vi "Update Low Limit.vi"(7 "Type":T1, 8 "error in (no error)":errorcluster, 9 "Low Limit":dbl, 10 "Channel Name":string, 11 "User BluelinesRedlines in":refnum<class "User BluelinesRedlines.lvclass">) -> (0 "error out":errorcluster, 3 "User BluelinesRedlines out":refnum<class "User BluelinesRedlines.lvclass">)   [LabVIEW 2020, in "VolatusGUIElements.lvlib" / "User BluelinesRedlines.lvclass"]
uses:
  User BluelinesRedlines.lvclass
  User BluelinesRedlines.lvclass/User BluelinesRedlines.ctl
  VolatusGUI/BluelinesRedlines Source/BLRL Type.ctl
  VolatusGUI/BluelinesRedlines Source/BluelinesRedlines Source.lvclass
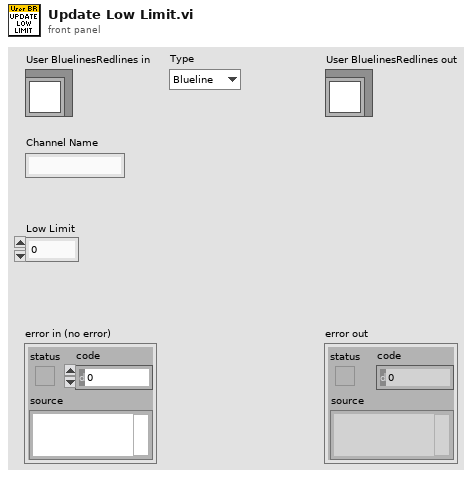
[diagram p1: front panel]
types:
  T1 = typedef "VolatusGUI.lvlib/BluelinesRedlines Source.lvclass/BLRL Type.ctl" = enum16{"Blueline", "Redline"}
  T2 = typedef "VolatusGUI.lvlib/BluelinesRedlines Source.lvclass/Range Limit Config.ctl" = cluster{"Channel":string, "Low Limit":dbl, "High Limit":dbl}
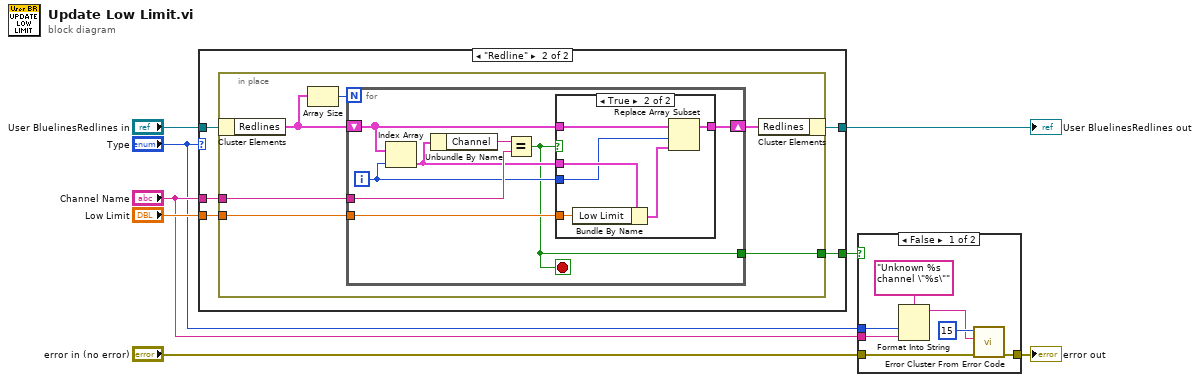
[diagram p0: block diagram]
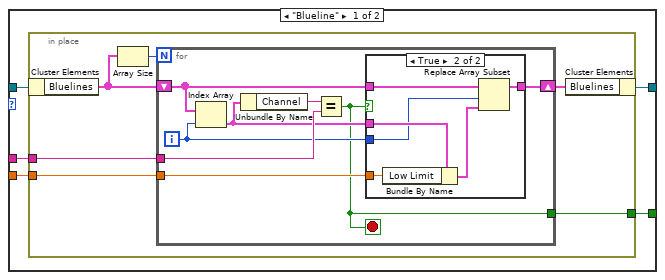
[diagram p3: hidden frame]
diagram:
  n1 = case shown="\"Redline\"" "Type" {
    tunnel: "User BluelinesRedlines in" -> [w13 w39]
    tunnel: [w12 w38] -> w7
    tunnel: "Channel Name" -> [w11 w37]
    tunnel: "Low Limit" -> [w10 w36]
    tunnel: [w9 w35] -> w5
    frame "Blueline" {
      n2 = in-place {
        in-place-border: w11 -> [w16]
        in-place-border: w10 -> [w15]
        in-place-border: [w14] -> w9
        n3 = in-place-cluster #1(w13) -> ("Bluelines"=w17:T2[])
        n4 = Array Size(array=w17) -> (size(s)=w18:i32)
        n5 = for {
          N: w18 -> [_]
          shift-right: [w21] -> w19
          shift-left: w17 -> [w25]
          tunnel: w16 -> [w26]
          tunnel: w15 -> [w24]
          tunnel: [w20] -> w14
          i -> [w23]
          stop <- w20 stop-if-true
          n6 = Index Array(array=w25, index=w23) -> (element=w22:T2)
          n7 = Unbundle By Name(w22) -> ("Channel"=w27:string)
          n8 = Equal?(x=w27, y=w26) -> (x = y?=w20:bool)
          n9 = case shown="True" w20 {
            tunnel: w25 -> [w28 w32]
            tunnel: w24 -> [_ w33]
            tunnel: w23 -> [_ w29]
            tunnel: w22 -> [_ w34]
            tunnel: [w28 w31] -> w21
            frame False {
            }
            frame True {
              n10 = Bundle By Name(cluster=w34, "Low Limit"=w33) -> (w30:T2)
              n11 = Replace Array Subset(array=w32, new element=w30, index=w29) -> (w31:T2[])
            }
          }
        }
        n12 = in-place-cluster #1("Bluelines"=w19) -> (w12:refnum<class "User BluelinesRedlines.lvclass">)
      }
    }
    frame "Redline" {
      n13 = in-place {
        in-place-border: w37 -> [w42]
        in-place-border: w36 -> [w41]
        in-place-border: [w40] -> w35
        n14 = in-place-cluster #2(w39) -> ("Redlines"=w43:T2[])
        n15 = Array Size(array=w43) -> (size(s)=w44:i32)
        n16 = for {
          N: w44 -> [_]
          shift-right: [w47] -> w45
          shift-left: w43 -> [w51]
          tunnel: w42 -> [w52]
          tunnel: w41 -> [w50]
          tunnel: [w46] -> w40
          i -> [w49]
          stop <- w46 stop-if-true
          n17 = Index Array(array=w51, index=w49) -> (element=w48:T2)
          n18 = Unbundle By Name(w48) -> ("Channel"=w53:string)
          n19 = Equal?(x=w53, y=w52) -> (x = y?=w46:bool)
          n20 = case shown="True" w46 {
            tunnel: w51 -> [w54 w58]
            tunnel: w50 -> [_ w59]
            tunnel: w49 -> [_ w55]
            tunnel: w48 -> [_ w60]
            tunnel: [w54 w57] -> w47
            frame False {
            }
            frame True {
              n21 = Bundle By Name(cluster=w60, "Low Limit"=w59) -> (w56:T2)
              n22 = Replace Array Subset(array=w58, new element=w56, index=w55) -> (w57:T2[])
            }
          }
        }
        n23 = in-place-cluster #2("Redlines"=w45) -> (w38:refnum<class "User BluelinesRedlines.lvclass">)
      }
    }
  }
  "User BluelinesRedlines out" <- w7
  n24 = case shown="False" w5 {
    tunnel: "error in (no error)" -> [w64 w68]
    tunnel: "Channel Name" -> [w67 _]
    tunnel: "Type" -> [w66 _]
    tunnel: [w61 w68] -> w1
    frame False {
      n25 = Format Into String(format string="Unknown %s channel \"%s\"", w66, w67) -> (resulting string=w62:string)  [unwired: 2 in, 1 out]
      n26 = call <vilib>:"Error Cluster From Error Code.vi"("error in (no error)"=w64, "error message (\"\")"=w62, "error code (0)"=15) -> ("error out"=w61:errorcluster)  [unwired: 6 in]
    }
    frame True {
    }
  }
  "error out" <- w1
